vi "sv_Update t0 (timestamp).vi"(7 "Reset Generation":bool, 9 "samples":i32, 10 "sample rate (S/s)":dbl format="%0.2f", 11 "tf previous":timestamp) -> (1 "dt":dbl, 2 "t0":timestamp, 3 "tf new":timestamp)   [LabVIEW 2017]
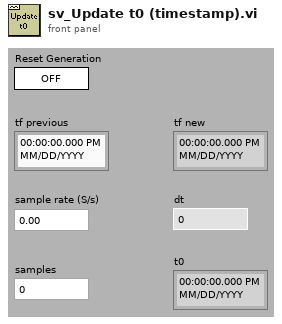
[diagram p1: front panel]
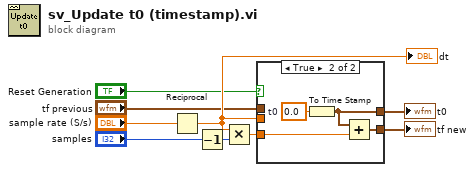
[diagram p0: block diagram]
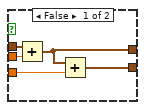
[diagram p2: hidden frame]
diagram:
  n1 = Reciprocal(x="sample rate (S/s)") -> (1/x=w7:dbl)
  "dt" <- w7
  n2 = Decrement(x="samples") -> (x-1=w3:i32)
  n3 = Multiply(x=w7, y=w3) -> (x*y=w4:dbl)
  n4 = case shown="True" "Reset Generation" {
    tunnel: "tf previous" -> [w14 _]
    tunnel: [w13 w17] -> w8
    tunnel: w7 -> [w11 _]
    tunnel: w4 -> [w10 w16]
    tunnel: [w12 w15] -> w2
    frame False {
      n5 = Add(x=w14, y=w11) -> (x+y=w13:timestamp)
      n6 = Add(x=w13, y=w10) -> (x+y=w12:timestamp)
    }
    frame True {
      w18 = 0.0  # t0
      n7 = To Time Stamp(1:w18) -> (0:w17:timestamp)
      n8 = Add(x=w17, y=w16) -> (x+y=w15:timestamp)
    }
  }
  "t0" <- w8
  "tf new" <- w2
